vi "Get SMO Address.vi"(8 "error in (no error)":errorcluster, 11 "Instrument.FrameworkTemplate":refnum<class "Instrument.FrameworkTemplate.lvclass">) -> (0 "error out":errorcluster, 2 "SMO Address":string, 3 "Instrument.FrameworkTemplate out":refnum<class "Instrument.FrameworkTemplate.lvclass">)   [LabVIEW 2019, in "Instrument.FrameworkTemplate.lvclass"]
uses:
  Instrument.FrameworkTemplate.lvclass
  <userlib>/LevyLab/Levylab Instruments/Instrument Types/VSource/Instrument.VSource.lvclass
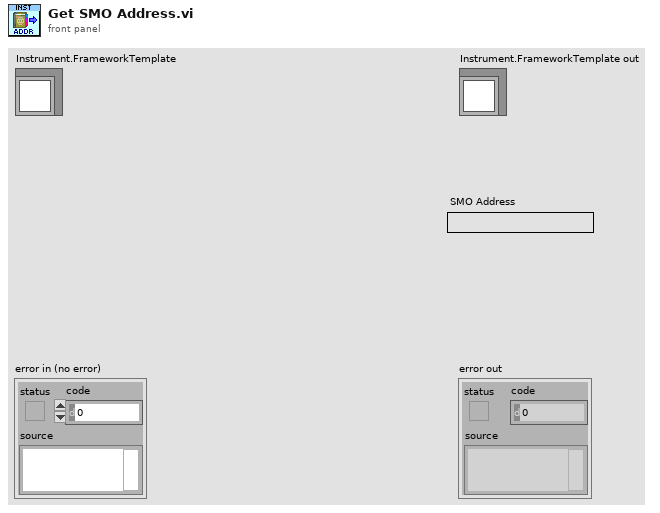
[diagram p1: front panel]
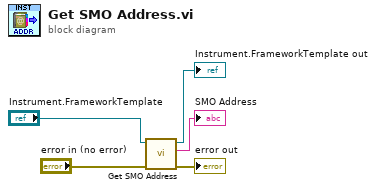
[diagram p0: block diagram]
diagram:
  n1 = call-parent "Get SMO Address.vi"("error in (no error)"="error in (no error)", "Instrument in"="Instrument.FrameworkTemplate") -> ("error out"=→"error out":errorcluster, "SMO Address"=→"SMO Address":string, "Instrument out"=→"Instrument.FrameworkTemplate out":refnum<class "Instrument.FrameworkTemplate.lvclass">)  [unwired: 7 in]
